vi "count.vi"(7 "count in":i32, 9 "fail count in":i32) -> (4 "count":string, 6 "fail count":string, 8 "Passrate":string, 10 "Fail Rate%":dbl)   [LabVIEW 2018]
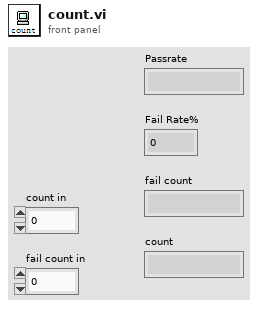
[diagram p1: front panel]
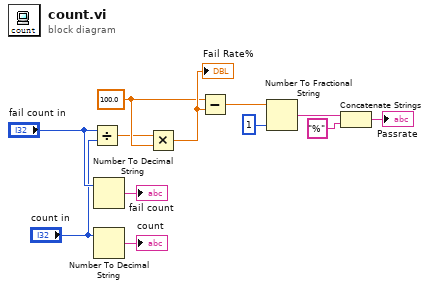
[diagram p0: block diagram]
diagram:
  w5 = 100.0 ("y")
  n1 = Divide(x="fail count in", y="count in") -> (x/y=w2:dbl)
  n2 = Number To Decimal String(number="fail count in") -> (decimal integer string=→"fail count":string)  [unwired: 1 out]
  n3 = Number To Decimal String(number="count in") -> (decimal integer string=→"count":string)  [unwired: 1 out]
  n4 = Multiply(x=w2, y=w5) -> (x*y=w6:dbl)
  "Fail Rate%" <- w6
  n5 = Subtract(x=w5, y=w6) -> (x-y=w7:dbl)
  n6 = Number To Fractional String(number=w7, precision (6)=i16 1 ("精度(6)")) -> (F-format string=w8:string)  [unwired: 2 out]
  n7 = Concatenate Strings(w8, "%") -> (→"Passrate":string)
